vi "RunExe-Wait For Target Ready.vi"(0 "Instance":u16, 7 "Timeout (s)":dbl=10.0 format="%#_13g", 11 "error in (no error)":errorcluster) -> (15 "error out":errorcluster)   [LabVIEW 2020]
doc: "We use a \"launcher\" VI with splash screen to start the main executable. This is not simply a matter of aesthetics; some exe's take a few seconds to become visible and a few seconds longer to become functional during which time it appears that nothing is happening. In contrast, the splash screen appears immediately.\n\nProblem: how do we know when the main exe is ready and the launcher can be terminated? Ideally, the launcher should determine that on its own and the main exe should have no knowledge of the launcher. In practice, I don't find a reliable way to detect that. \n\nRejected solutions: the launcher could be part of the main VI, but that functionality doesn't really belong there. The launcher could load and run the main VI (in a single exe), but that the loading of the main VI from an exe is messy. Also, the main exe should stand on its own.\n\nSolution: we'll have the main exe broadcast one time over a socket that it is ready. It should not be an error if no one is listening for the broadcast.\n\nThis VI is used by the launcher to listen for that broadcast."
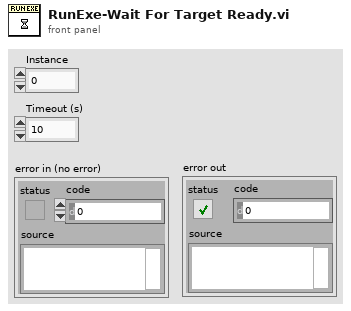
[diagram p1: front panel]
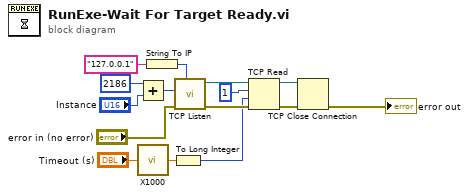
[diagram p0: block diagram]
diagram:
  n1 = Add(x=u16 2186 ("port"), y="Instance") -> (x+y=w2:u16)
  n2 = call "X1000.vi"("X"="Timeout (s)") -> ("X/1000"=w8:dbl)
  n3 = String To IP(1:"127.0.0.1" ("name")) -> (0:w13:u32)
  n4 = To Long Integer(number=w8) -> (32bit integer=w7:i32)
  n5 = call <vilib>:"TCP Listen.vi"("net address"=w13, "error in (no error)"="error in (no error)", "port"=w2) -> ("error out"=w10:errorcluster, "connection ID"=w11:refnum<k5>)  [unwired: 4 in, 3 out]
  n6 = TCP Read(connection ID=w11, bytes to read=1, error in (no error)=w10, 9:w7) -> (connection ID out=w4:refnum<k5>, error out=w5:errorcluster)  [unwired: 1 in, 1 out]
  n7 = TCP Close Connection(connection ID=w4, error in (no error)=w5) -> (error out=→"error out":errorcluster)  [unwired: 1 in, 1 out]
